vi "ACC_LabVIEW_Disconnect.vi"(0 "DeviceReferenceIn":cluster{"ID":u32}, 3 "return error strings buffer size (Byte)":u32=500, 5 "error in (no error)":errorcluster) -> (19 "error out":errorcluster)   [LabVIEW 2014, in "ACC_LabVIEW.lvlib"]
doc: "Perform a \"read\" inside the GSI - accelerator control system."
uses:
  ACC_LabVIEW.lvlib
  lib/ACC_Interface_Wrapper.dll
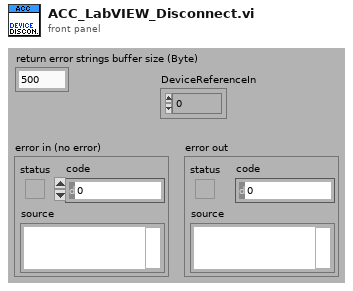
[diagram p1: front panel]
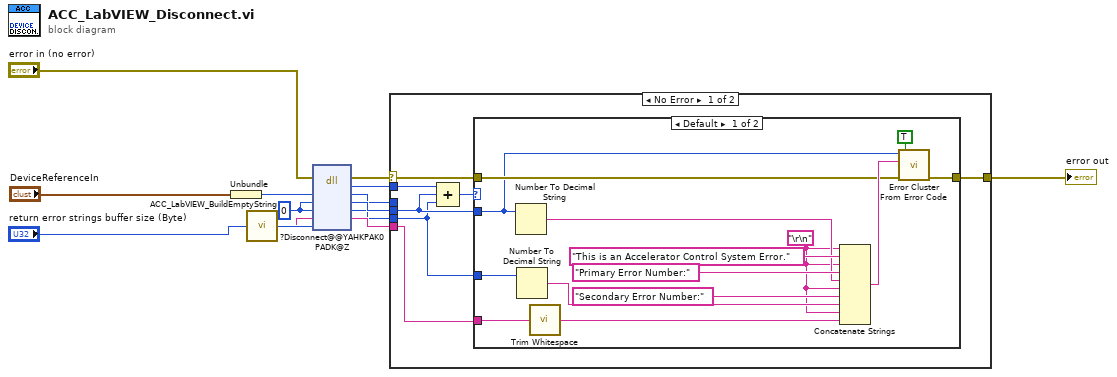
[diagram p0: block diagram]
diagram:
  w4 = u32 0 ("no input, only output")
  n1 = Unbundle("DeviceReferenceIn") -> ("ID"=w1:u32)
  n2 = call "ACC_LabVIEW_BuildEmptyString.vi"("Length"="return error strings buffer size (Byte)") -> ("String"=w10:string)
  n3 = dll-call lib="D:/Git/CS-framework/CSinstr.lib/ACC_LabVIEW_Interface/lib/ACC_Interface_Wrapper.dll" fn="?Disconnect@@YAHKPAK0PADK@Z"(error in="error in (no error)", "DeviceHandle"=w1, "ErrPrimStat"=w4, "ErrSecStat"=w4, "ErrorMSG"=w10, "ErrorMSG_Size"="return error strings buffer size (Byte)") -> (error out=w9:errorcluster, "ErrorPrimState"=w8:i32, "DeviceHandle"=w3:u32, "ErrPrimStat"=w6:u32, "ErrSecStat"=w5:u32, "ErrorMSG"=w7:string)  [unwired: 3 in, 1 out]
  n4 = case shown="No Error" w9 {
    selector: w9 -> [w18 w36]
    tunnel: w8 -> [w20 _]
    tunnel: [w15 w36] -> w12
    tunnel: w7 -> [w14 _]
    tunnel: w6 -> [w17 _]
    tunnel: w5 -> [w16 _]
    tunnel: w3 -> [_ _]
    frame No Error {
      n5 = Compound Arithmetic op=ADD(w20, w17, w16) -> (w19:u32)
      n6 = case shown="Default" w19 {
        tunnel: w18 -> [w24 w35]
        tunnel: w17 -> [w22 _]
        tunnel: w16 -> [w34 _]
        tunnel: [w23 w35] -> w15
        tunnel: w14 -> [w28 _]
        frame Default {
          w26 = "\r\n"
          n7 = Number To Decimal String(number=w22) -> (decimal integer string=w31:string)  [unwired: 1 in]
          n8 = Number To Decimal String(number=w34) -> (decimal integer string=w29:string)  [unwired: 1 in]
          n9 = call <vilib>:"Trim Whitespace.vi"("string"=w28) -> ("trimmed string"=w27:string)  [unwired: 1 in]
          n10 = Concatenate Strings(w26, "This is an Accelerator Control System Error.", w26, "Primary Error Number:", w31, w26, "Secondary Error Number:", w29, w26, w27) -> (w25:string)
          n11 = call <vilib>:"Error Cluster From Error Code.vi"("show call chain? (False)"=TRUE, "error in (no error)"=w24, "error message (\"\")"=w25, "error code (0)"=w22) -> ("error out"=w23:errorcluster)  [unwired: 5 in]
        }
        frame 0 {
          # "no error"
        }
      }
    }
    frame Error {
    }
  }
  "error out" <- w12
